vi "Find Port.vi"(8 "error in":errorcluster, 10 "port number":u16, 11 "Ballard MIL-STD 1553 custom device in":T1 format="%.0x") -> (0 "error out":errorcluster, 2 "port":T1 format="%.0x", 3 "Ballard MIL-STD 1553 custom device out":T1 format="%.0x", 4 "found?":bool)   [LabVIEW 2020, in "AIM MIL-STD-1553 Scripting.lvlib"]
doc: "Within the specified <b>Ballard MIL-STD-1553 custom device in</b>, searches for an instance of a port with matching <b>port number</b>. If a match is found, returns the matching <b>port</b> reference. If no match is found, the returned reference is invalid and <b>found?</b> equals False."
uses:
  AIM MIL-STD-1553 Scripting.lvlib
  <vilib>/NI VeriStand/Custom Device API/Custom Device Item Ref.ctl
  <vilib>/NI VeriStand/Custom Device API/Custom Device API.lvlib
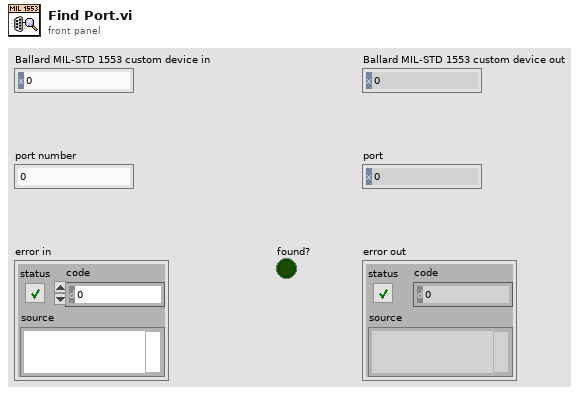
[diagram p1: front panel]
types:
  T1 = typedef "Custom Device API.lvlib/Custom Device Item Ref.ctl" = u64
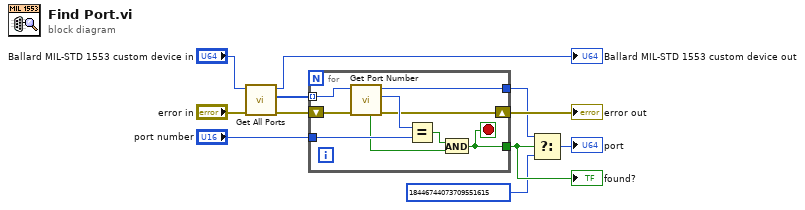
[diagram p0: block diagram]
diagram:
  n1 = call "Get All Ports.vi"("error in"="error in", "Ballard MIL-STD 1553 custom device in"="Ballard MIL-STD 1553 custom device in") -> ("error out"=w6:errorcluster, "ports"=w9:T1[], "Ballard MIL-STD 1553 custom device out"=→"Ballard MIL-STD 1553 custom device out":T1)  [unwired: 7 in]
  n2 = for {
    tunnel: w9 -> [w20] mode=indexing
    tunnel: "port number" -> [w19]
    tunnel: [w13] -> w3
    tunnel: [w12] -> w4
    shift-right: [w14] -> w5
    shift-left: w6 -> [w15]
    stop <- w12 stop-if-true
    n3 = call "Get Port Number.vi"("error in"=w15, "port in"=w20) -> ("error out"=w14:errorcluster, "port number"=w18:u16, "port out"=w13:T1, "found?"=w17:bool)  [unwired: 6 in]
    n4 = Equal?(x=w18, y=w19) -> (x = y?=w16:bool)
    n5 = And(x=w16, y=w17) -> (x .and. y?=w12:bool)
  }
  "error out" <- w5
  "found?" <- w4
  n6 = Select(t=w3, s=w4, f=T1 18446744073709551615 ("Invalid Ref")) -> (s? t:f=→"port":T1)
